vi "RM.checkReservation.vi"(5 "Resource Type":T1, 7 "Direction":T2, 8 "error in":errorcluster, 10 "name in bitfile":string, 11 "reservation DB in":variant) -> (0 "error out":errorcluster, 2 "found?":bool, 3 "reservation DB out":variant)   [LabVIEW 2016, in "FPGA Addon Shared.lvlib"]
uses:
  FPGA Addon Shared.lvlib
  RM.resourceDirection.ctl
  RM.resourceType.ctl
panel:
  out "reserver":string
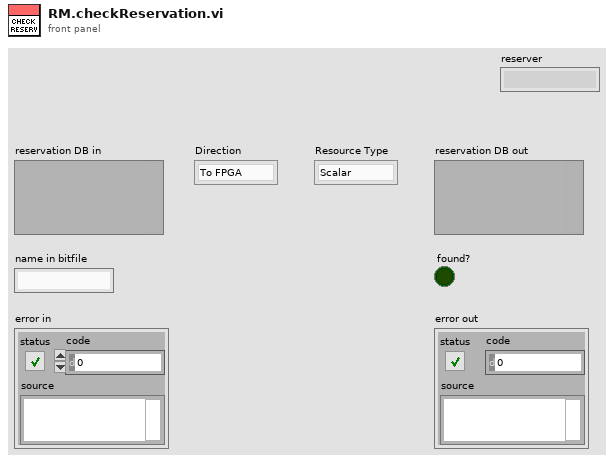
[diagram p1: front panel]
types:
  T1 = typedef "FPGA Addon Shared.lvlib/RM.resourceType.ctl" = enum16{"Scalar", "Waveform"}
  T2 = typedef "FPGA Addon Shared.lvlib/RM.resourceDirection.ctl" = enum16{"To FPGA", "From FPGA"}
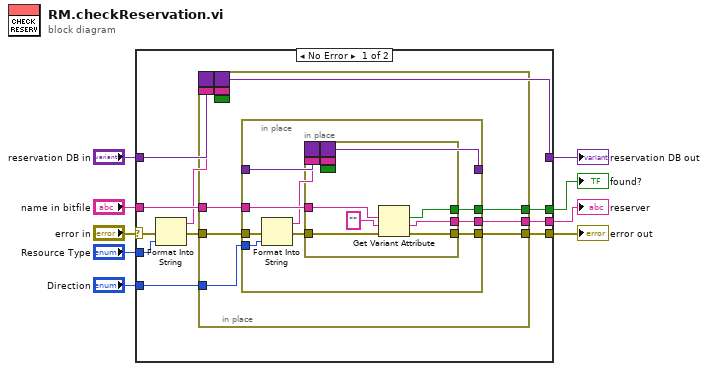
[diagram p0: block diagram]
diagram:
  n1 = case shown="No Error" "error in" {
    selector: "error in" -> [w13 w47]
    tunnel: "reservation DB in" -> [w20 w48]
    tunnel: "Direction" -> [w19 _]
    tunnel: [w18 w48] -> w2
    tunnel: "name in bitfile" -> [w17 _]
    tunnel: "Resource Type" -> [w16 _]
    tunnel: [w12 w47] -> w4
    tunnel: [w11 _] -> w3
    tunnel: [w10 _] -> w1
    frame No Error {
      n2 = Format Into String(error in=w13, w16) -> (resulting string=w15:string, error out=w14:errorcluster)  [unwired: 2 in]
      n3 = in-place {
        in-place-border: w19 -> [w28]
        in-place-border: w17 -> [w25]
        in-place-border: w14 -> [w24]
        in-place-border: [w23] -> w12
        in-place-border: [w22] -> w11
        border: w20 -> [_]
        border: w15 -> [_]
        border: [_] -> w18
        border: _ -> [_]
        border: _ -> [_]
        in-place-border: [w21] -> w10
        n4 = in-place {
          in-place-border: w28 -> [w35]
          in-place-border: w27 -> [w38]
          in-place-border: [w37] -> w26
          in-place-border: w25 -> [w36]
          in-place-border: w24 -> [w33]
          in-place-border: [w31] -> w23
          in-place-border: [w30] -> w22
          in-place-border: [w29] -> w21
          n5 = Format Into String(error in=w33, w35) -> (resulting string=w34:string, error out=w32:errorcluster)  [unwired: 2 in]
          n6 = in-place {
            in-place-border: w36 -> [w42]
            in-place-border: w32 -> [w45]
            in-place-border: [w44] -> w31
            in-place-border: [w43] -> w30
            border: w38 -> [_]
            border: w34 -> [_]
            border: [_] -> w37
            border: _ -> [_]
            border: _ -> [_]
            in-place-border: [w39] -> w29
            n7 = Get Variant Attribute(Variant=w41, name=w42, default value (empty Variant)="" ("name in bitfile"), error in=w45) -> (duplicate Variant=w46:variant, found=w43:bool, value=w39:string, error out=w44:errorcluster)
          }
        }
      }
    }
    frame Error {
    }
  }
  "reservation DB out" <- w2
  "error out" <- w4
  "found?" <- w3
  "reserver" <- w1
